vi "Delete_Data_Core.vi"(8 "error in":errorcluster, 11 "Data In":T1={"vector_qdrant"=refnum, "llm_openai"=refnum, "llm_openai_embedding"=refnum, "simple_html_chat_ui"=refnum}) -> (0 "error out":errorcluster)   [LabVIEW 2020]
uses:
  Type Defs/Data_Core.ctl
  src/vectorstore/vector_qdrant/vector_qdrant.lvclass
  src/models/llm_openai_chatmodels/llm_openai_chatmodels.lvclass
  src/models/llm_openai_embedding/llm_openai_embedding.lvclass
  src/user_interfaces/simple_html_chat_ui/simple_html_chat_ui.lvclass
  Dependencies/WebSockets-API/Source/WebSockets/WebSocket Server/WebSocket Server.lvclass
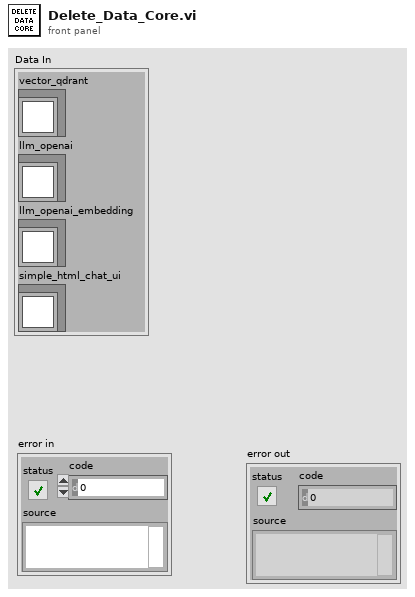
[diagram p1: front panel]
types:
  T1 = typedef "Data_Core.ctl" = cluster{"vector_qdrant":refnum<class "vector_qdrant.lvclass">, "llm_openai":refnum<class "llm_openai_chatmodels.lvclass">, "llm_openai_embedding":refnum<class "llm_openai_embedding.lvclass">, "simple_html_chat_ui":refnum<class "simple_html_chat_ui.lvclass">}
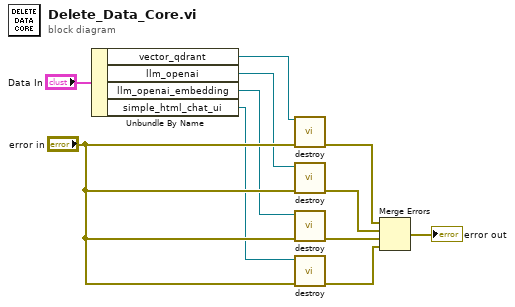
[diagram p0: block diagram]
diagram:
  n1 = Unbundle By Name("Data In") -> ("vector_qdrant"=w1:refnum<class "vector_qdrant.lvclass">, "llm_openai"=w2:refnum<class "llm_openai_chatmodels.lvclass">, "llm_openai_embedding"=w3:refnum<class "llm_openai_embedding.lvclass">, "simple_html_chat_ui"=w4:refnum<class "simple_html_chat_ui.lvclass">)
  n2 = call-dynamic "destroy.vi"("vector_qdrant in"=w1, "error in (no error)"="error in") -> ("error out"=w7:errorcluster)  [unwired: 12 in, 1 out]
  n3 = call-dynamic "destroy.vi"("error in (no error)"="error in", "abstract_llm_base in"=w2) -> ("error out"=w8:errorcluster)  [unwired: 8 in, 1 out]
  n4 = call-dynamic "destroy.vi"("error in (no error)"="error in", "llm_openai_embedding in"=w3) -> ("error out"=w9:errorcluster)  [unwired: 8 in, 1 out]
  n5 = call "destroy.vi"("error in (no error)"="error in", "simple_html_chat_ui in"=w4) -> ("error out"=w10:errorcluster)  [unwired: 8 in, 1 out]
  n6 = Merge Errors(w7, w8, w9, w10) -> (→"error out":errorcluster)
